vi "Send Decrement Multi Instrument Handler.vi"(10 "Hander Index":i32, 11 "Message Enqueuer":refnum<class "Message Enqueuer.lvclass">) -> (0 "error out":errorcluster)   [LabVIEW 2020, in "Instrument Handler.lvlib" / "Decrement Multi Instrument Handler Msg.lvclass"]
doc: "This VI sends the message to the Instrument Handler with High priority."
uses:
  Decrement Multi Instrument Handler Msg.lvclass
  PPL/HDH.Actor Framework.Core.Actor.lvlibp/1abvi3w/vi.lib/ActorFramework/Message Enqueuer/Message Enqueuer.lvclass
  PPL/HDH.Actor Framework.Core.Actor.lvlibp/1abvi3w/vi.lib/ActorFramework/Message Enqueuer/Message Priority.ctl
  Decrement Multi Instrument Handler Msg.lvclass/Decrement Multi Instrument Handler Msg.ctl
  C:/Current projects/WS/PPL/HDH.Actor Framework.Core.Actor.lvlibp/1abvi3w/vi.lib/ActorFramework/Message/Message.lvclass
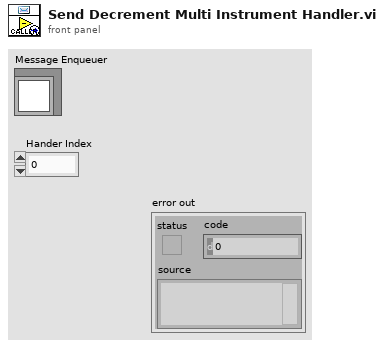
[diagram p1: front panel]
types:
  T1 = typedef "HDH.Actor Framework.Core.Actor.lvlibp/Message Enqueuer.lvclass/Message Priority.ctl" = enum16{"Low", "Normal", "High"}
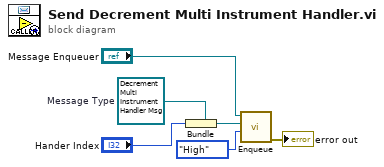
[diagram p0: block diagram]
diagram:
  w4 = refnum<class "Decrement Multi Instrument Handler Msg.lvclass"> refnum  # Message Type
  n1 = Bundle(cluster=w4, "Hander Index") -> (w3:refnum<class "Decrement Multi Instrument Handler Msg.lvclass">)
  n2 = call "Enqueue.vi"("Message Priority (Normal)"=Message_Priority."High", "Message"=w3, "Message Enqueuer in"="Message Enqueuer") -> ("error out"=→"error out":errorcluster)  [unwired: 7 in, 1 out]
